vi "Set Input Configuration File Path.vi"(8 "error in (no error)":errorcluster, 11 "configuration file":path) -> (0 "error out":errorcluster)   [LabVIEW 2022 SP3, in "Config Dialog.lvlib"]
uses:
  Config Dialog.lvlib
  audio settings.ctl
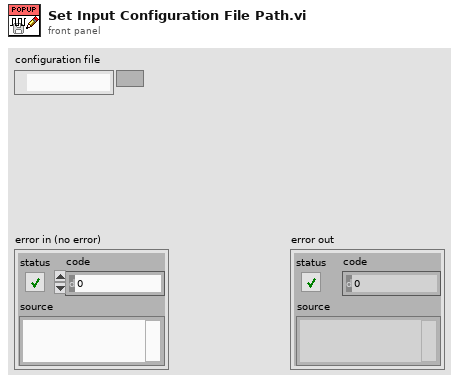
[diagram p1: front panel]
types:
  T1 = typedef "Config Dialog.lvlib/audio settings.ctl" = cluster{"input cfg file":string}
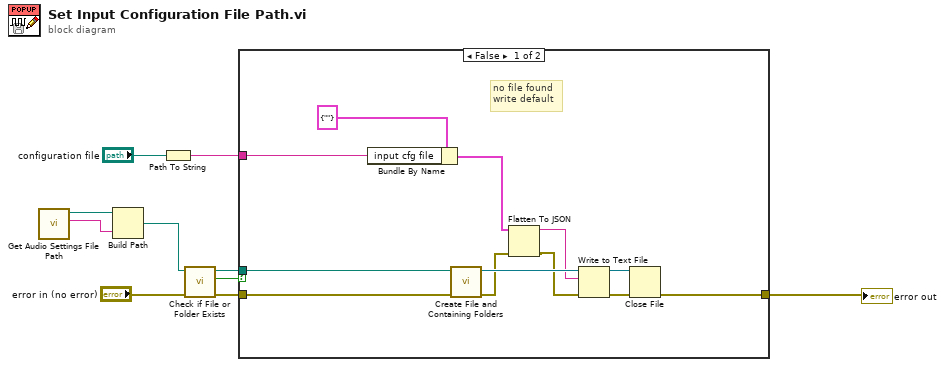
[diagram p0: block diagram]
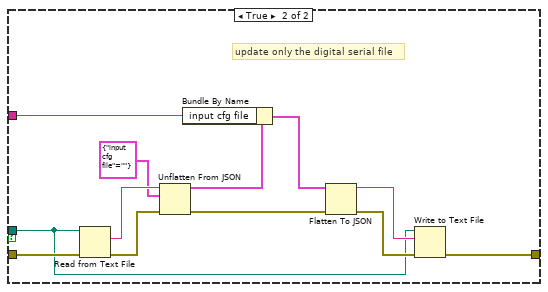
[diagram p2: hidden frame]
diagram:
  n1 = call "Get Audio Settings File Path.vi"() -> ("file name"=w5:string, "directory"=w6:path)  [unwired: 10 in]
  n2 = Build Path(base path=w6, name or relative path=w5) -> (appended path=w4:path)
  n3 = Path To String(path="configuration file") -> (string=w1:string)
  n4 = call <vilib>:"Check if File or Folder Exists.vi"("error in (no error)"="error in (no error)", "path"=w4) -> ("error out"=w10:errorcluster, "file or folder exists?"=w9:bool, "dup path"=w8:path)  [unwired: 7 in]
  n5 = case shown="False" w9 {
    tunnel: w10 -> [w22 w25]
    tunnel: w8 -> [w21 w24]
    tunnel: [w18 w23] -> w3
    tunnel: w1 -> [w11 w30]
    frame False {
      # "no file found\nwrite default"
      n6 = Bundle By Name(cluster=T1 {"input cfg file"=""} ("audio settings"), "input cfg file"=w11) -> (w12:T1)
      n7 = call <vilib>:"Create File and Containing Folders.vi"("error in (no error)"=w22, "file path"=w21) -> ("error out"=w16:errorcluster, "refnum out"=w17:refnum<file>)  [unwired: 8 in]
      n8 = Flatten To JSON(anything=w12, error in (no error)=w16) -> (JSON string=w14:string, 11:w15:errorcluster)  [unwired: 1 in]
      n9 = Write to Text File(file (use dialog)=w17, text=w14, error in=w15) -> (refnum out=w19:refnum<file>, error out=w20:errorcluster)  [unwired: 1 in, 1 out]
      n10 = Close File(refnum=w19, error in=w20) -> (error out=w18:errorcluster)  [unwired: 1 out]
    }
    frame True {
      # "update only the digital serial file"
      n11 = Read from Text File(file (use dialog)=w24, error in=w25) -> (text=w33:string, error out=w34:errorcluster)  [unwired: 2 in, 2 out]
      n12 = Unflatten From JSON(JSON string=w33, type and defaults=T1 {"input cfg file"=""} ("audio settings"), error in (no error)=w34) -> (value=w31:T1, error out=w29:errorcluster)  [unwired: 4 in]
      n13 = Bundle By Name(cluster=w31, "input cfg file"=w30) -> (w28:T1)
      n14 = Flatten To JSON(anything=w28, error in (no error)=w29) -> (JSON string=w26:string, 11:w27:errorcluster)  [unwired: 1 in]
      n15 = Write to Text File(file (use dialog)=w24, text=w26, error in=w27) -> (error out=w23:errorcluster)  [unwired: 1 in, 2 out]
    }
  }
  "error out" <- w3
